vi "Categorize lvclass and other files.vi"(8 "error in (no error)":errorcluster, 11 "Created Files":path[](array[path])) -> (0 "error out":errorcluster, 1 "Other Files":path[](array[path]), 2 "LVClass Files":path[](array[path]))   [LabVIEW 2020, in "Mock Class Updater.lvclass"]
uses:
  Mock Class Updater.lvclass
  Mock Class Updater.lvclass/Mock Class Updater.ctl
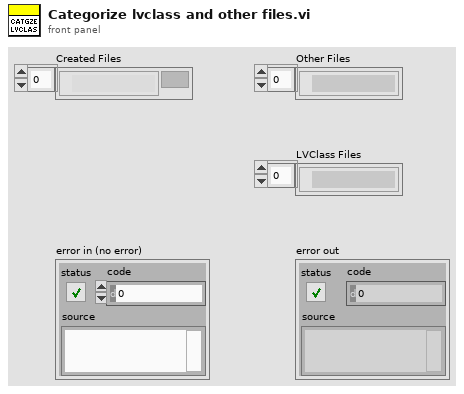
[diagram p1: front panel]
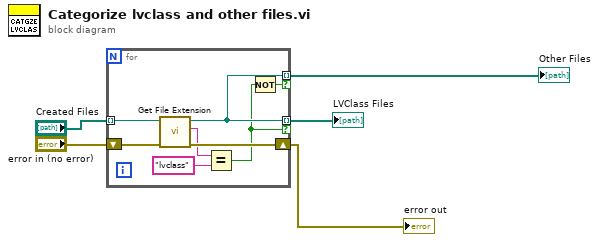
[diagram p0: block diagram]
diagram:
  n1 = for {
    tunnel: "Created Files" -> [w13] mode=indexing
    shift-right: [w11] -> w3
    shift-left: "error in (no error)" -> [w12]
    tunnel: [w8] -> w4 mode=indexing if=w7
    tunnel: [w8] -> w5 mode=indexing if=w6
    n2 = call <vilib>:"Get File Extension.vi"("error in (no error)"=w12, "file"=w13) -> ("error out"=w11:errorcluster, "lowercase file extension"=w10:string, "dup file"=w8:path)  [unwired: 5 in, 2 out]
    n3 = Equal?(x=w10, y="lvclass") -> (x = y?=w7:bool)
    n4 = Not(x=w7) -> (.not. x?=w6:bool)
  }
  "Other Files" <- w5
  "LVClass Files" <- w4
  "error out" <- w3
